vi "serialreadv1.vi"() -> ()   [LabVIEW 2019]
doc: "This example performs a serial port write and a serial port read. The parameters set for the serial port must match the parameters of the connected instrument or device. The VISA Configure Serial Port VI sets the configuration parameters. The front panel displays the controls used to configure the basic parameters, such as baud rate, data bits, and parity. The VI passes the VISA resource name to other VIs that perform operations on that VISA resource. The VISA Write function sends a command to the serial device and the VISA Read function returns data based on the command. The VISA Close function then closes the reference to the serial device. It is important to close the reference; otherwise, further communication through that port might not be possible."
uses:
  support/Serial - Settings.ctl
  <vilib>/Instr/_visa.llb/VISA Configure Serial Port (Instr).vi
panel:
  out "Serial Settings:Wire Mode":i16(ring)=128 items=["Unknown"=-1, "RS485/Wire4"=0, "RS485/Wire2-EchoDTR"=1, "RS485/Wire2-CtrlDTR"=2, "RS485/Wire2-Auto"=3, "RS232/DTE"=128, "RS232/DCE"=129, "RS232/Auto"=130]
  out "message":string="Error -1073807339 occurred at VISA Read in Simple Serial one hex message.vi\r\n\r\nPossible reason(s):\n\r\nVISA:  (Hex 0xBFFF0015) Timeout expired before operation completed."
  out "Read Buffer in Normal":string
  in  "Enable Termination\nChar (T)":bool=TRUE
  in  "termination char\n(0xA = '\\n' = LF)":u8=13 format="%.0x"
  out "return count 2":u32
  out "Read Buffer in Hex":string
  in  "Message in Hex":string="\u0002\u0003I\u0015\u0000\u0001ƒ’"
  in  "Serial Settings":T1={"baud rate"=9600, "data bits"=8, "parity"=enum."Even", "stop bits"=10, "flow control"=0} {"flow control" items=["None"=0, "XON/XOFF"=1, "RTS/CTS"=2, "DTR/DSR"=4]; "stop bits" items=["1.0"=10, "1.5"=15, "2.0"=20]; "data bits" min=5 max=8 step=1; "baud rate" items=["75"=75, "110"=110, "134"=134, "150"=150, "300"=300, "600"=600, "1200"=1200, "1800"=1800, "2400"=2400, "4800"=4800, "7200"=7200, "9600"=9600, "14400"=14400, "19200"=19200, "28800"=28800, "38400"=38400, "56000"=56000, "57600"=57600, "115200"=115200, "128000"=128000, "230400"=230400]}
  in  "VISA resource name":refnum<visa-resource-name>="COM6"
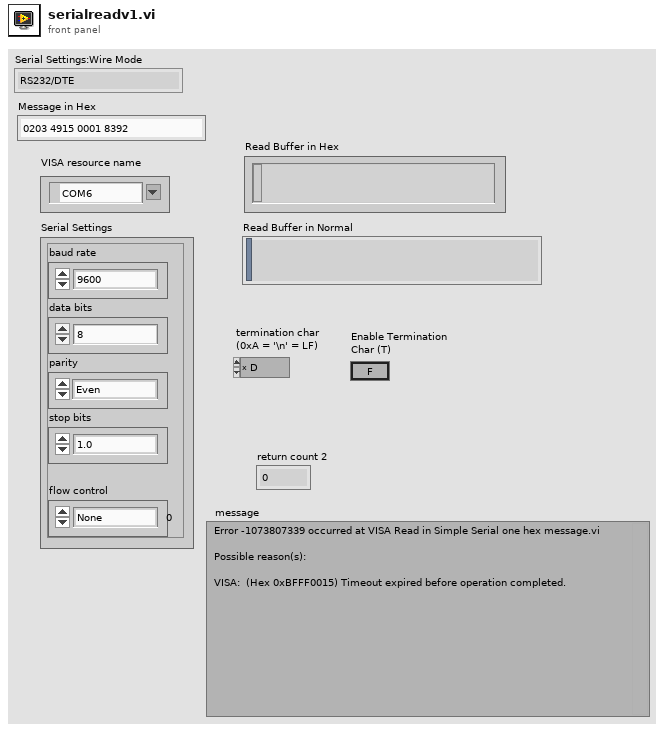
[diagram p1: front panel]
types:
  T1 = typedef "Serial - Settings.ctl" = cluster{"baud rate":u32, "data bits":u16, "parity":enum16{"None", "Odd", "Even", "Mark", "Space"}, "stop bits":u16, "flow control":u16}
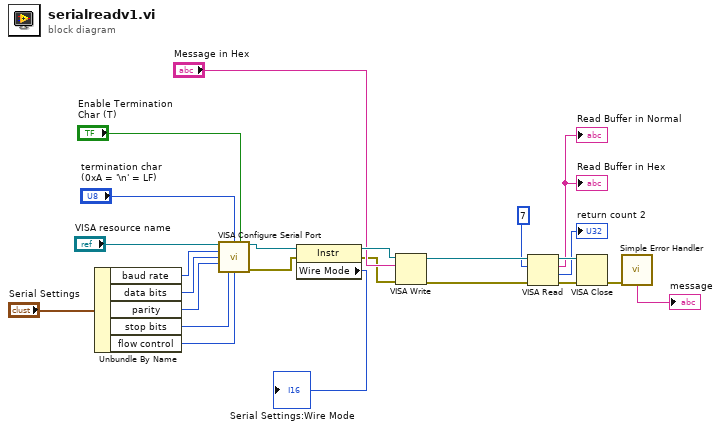
[diagram p0: block diagram]
diagram:
  n1 = Unbundle By Name("Serial Settings") -> ("baud rate"=w10:u32, "data bits"=w18:u16, "parity"=w17:enum16{"None", "Odd", "Even", "Mark", "Space"}, "stop bits"=w16:u16, "flow control"=w15:u16)
  n2 = call-poly "VISA Configure Serial Port"("VISA resource name"="VISA resource name", "termination char\n(0xA = '\\n' = LF)"="termination char\n(0xA = '\\n' = LF)", "Enable Termination\nChar (T)"="Enable Termination\nChar (T)", "baud rate (9600)"=w10, "data bits (8)"=w18, "parity (0:none)"=w17, "stop bits (10: 1 bit)"=w16, "flow control (0:none)"=w15) -> ("VISA resource name out"=w9:refnum<visa-resource-name>, "error out"=w7:errorcluster)  [unwired: 2 in, 4 out]
  n3 = property class="Instr"(reference=w9, error in=w7) -> (reference out=w8:refnum<visa-resource-name>, error out=w4:errorcluster, "Wire Mode"=→"Serial Settings:Wire Mode":i16)
  n4 = VISA Write(VISA resource name=w8, write buffer="Message in Hex", error in (no error)=w4) -> (VISA resource name out=w3:refnum<visa-resource-name>, error out=w1:errorcluster)  [unwired: 1 out]
  n5 = VISA Read(VISA resource name=w3, byte count=u32 7, error in (no error)=w1) -> (VISA resource name out=w22:refnum<visa-resource-name>, read buffer=→"Read Buffer in Hex" →"Read Buffer in Normal":string, return count=→"return count 2":u32, error out=w23:errorcluster)
  n6 = VISA Close(VISA resource name=w22, error in (no error)=w23) -> (error out=w21:errorcluster)
  n7 = call <vilib>:"Simple Error Handler.vi"("error in (no error)"=w21) -> ("message"=→"message":string)  [unwired: 1 in, 7 out]
